vi "Acquire.vi"(5 "Weight Port":refnum<visa-resource-name>, 6 "error in":errorcluster, 7 "GlobalData":T1, 8 "Calibration":variant, 9 "Salinity":refnum<k21>, 10 "Temperature":refnum<k21>, 11 "Pressure":refnum<k21>) -> (0 "Weight Port":refnum<visa-resource-name>, 1 "Salinity":refnum<k21>, 2 "Temperature":refnum<k21>, 3 "Pressure":refnum<k21>, 4 "error out":errorcluster)   [LabVIEW 2024]
uses:
  <vilib>/DAQmx/read.llb/DAQmx Read (Analog DBL 1Chan 1Samp).vi
  controls/GlobalData.ctl
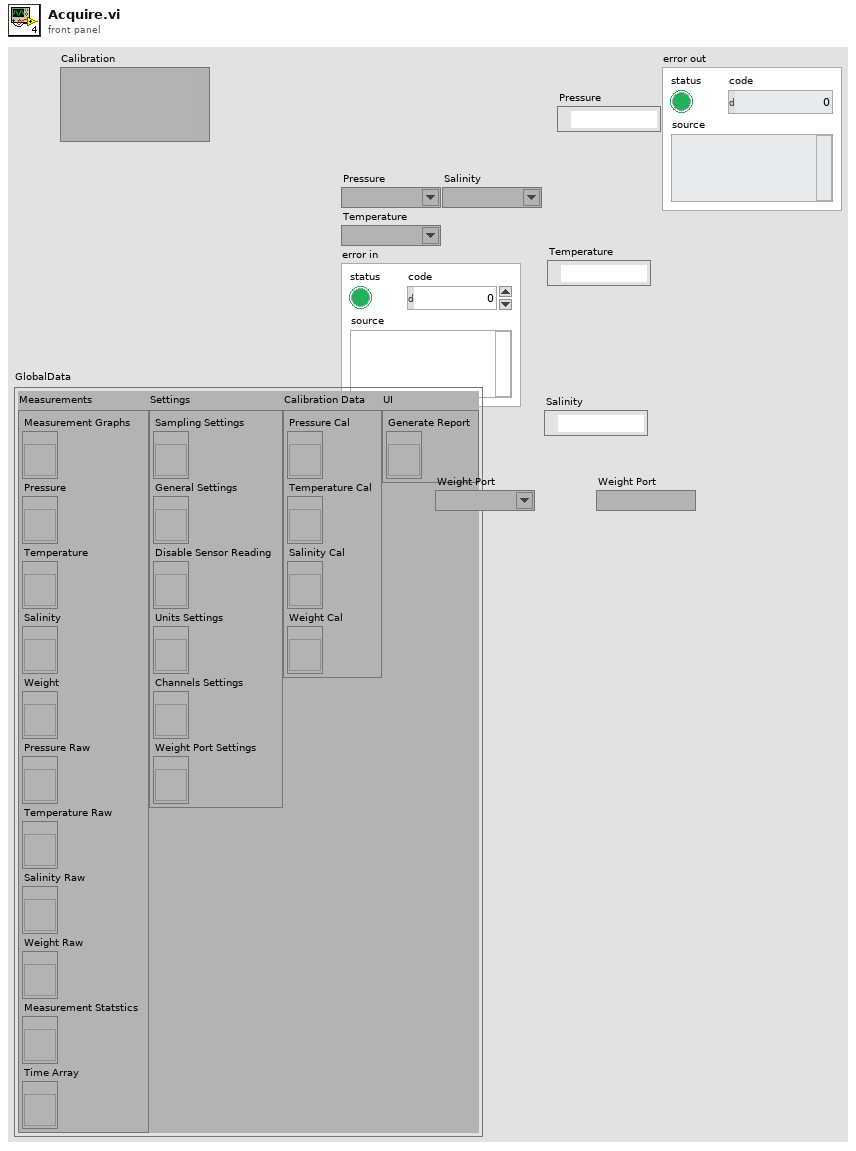
[diagram p1: front panel]
types:
  T1 = typedef "GlobalData.ctl" = cluster{"Measurements":cluster{"Measurement Graphs":refnum<vi>, "Pressure":refnum<vi>, "Temperature":refnum<vi>, "Salinity":refnum<vi>, "Weight":refnum<vi>, "Pressure Raw":refnum<vi>, "Temperature Raw":refnum<vi>, "Salinity Raw":refnum<vi>, "Weight Raw":refnum<vi>, "Measurement Statstics":refnum<vi>, "Time Array":refnum<vi>}, "Settings":cluster{"Sampling Settings":refnum<vi>, "General Settings":refnum<vi>, "Disable Sensor Reading":refnum<vi>, "Units Settings":refnum<vi>, "Channels Settings":refnum<vi>, "Weight Port Settings":refnum<vi>}, "Calibration Data":cluster{"Pressure Cal":refnum<vi>, "Temperature Cal":refnum<vi>, "Salinity Cal":refnum<vi>, "Weight Cal":refnum<vi>}, "UI":cluster{"Generate Report":refnum<vi>}}
  T2 = typedef "Units.ctl" = cluster{"Pressure":enum16{"PSI", "Bar", "atm", "Pa"}, "Temperature":enum16{"C", "K", "F"}, "Salinity":enum16{"ppm", "ppt", "PSU"}, "Weight":enum16{"Kg", "g", "oz", "ib"}}
  T3 = cluster{"C (Y-Intercept)":dbl, "M (Gradient)":dbl}
  T4 = cluster{"Pressure":dbl[], "Temperature":dbl[], "Salinity":dbl[], "Weight":dbl[]}
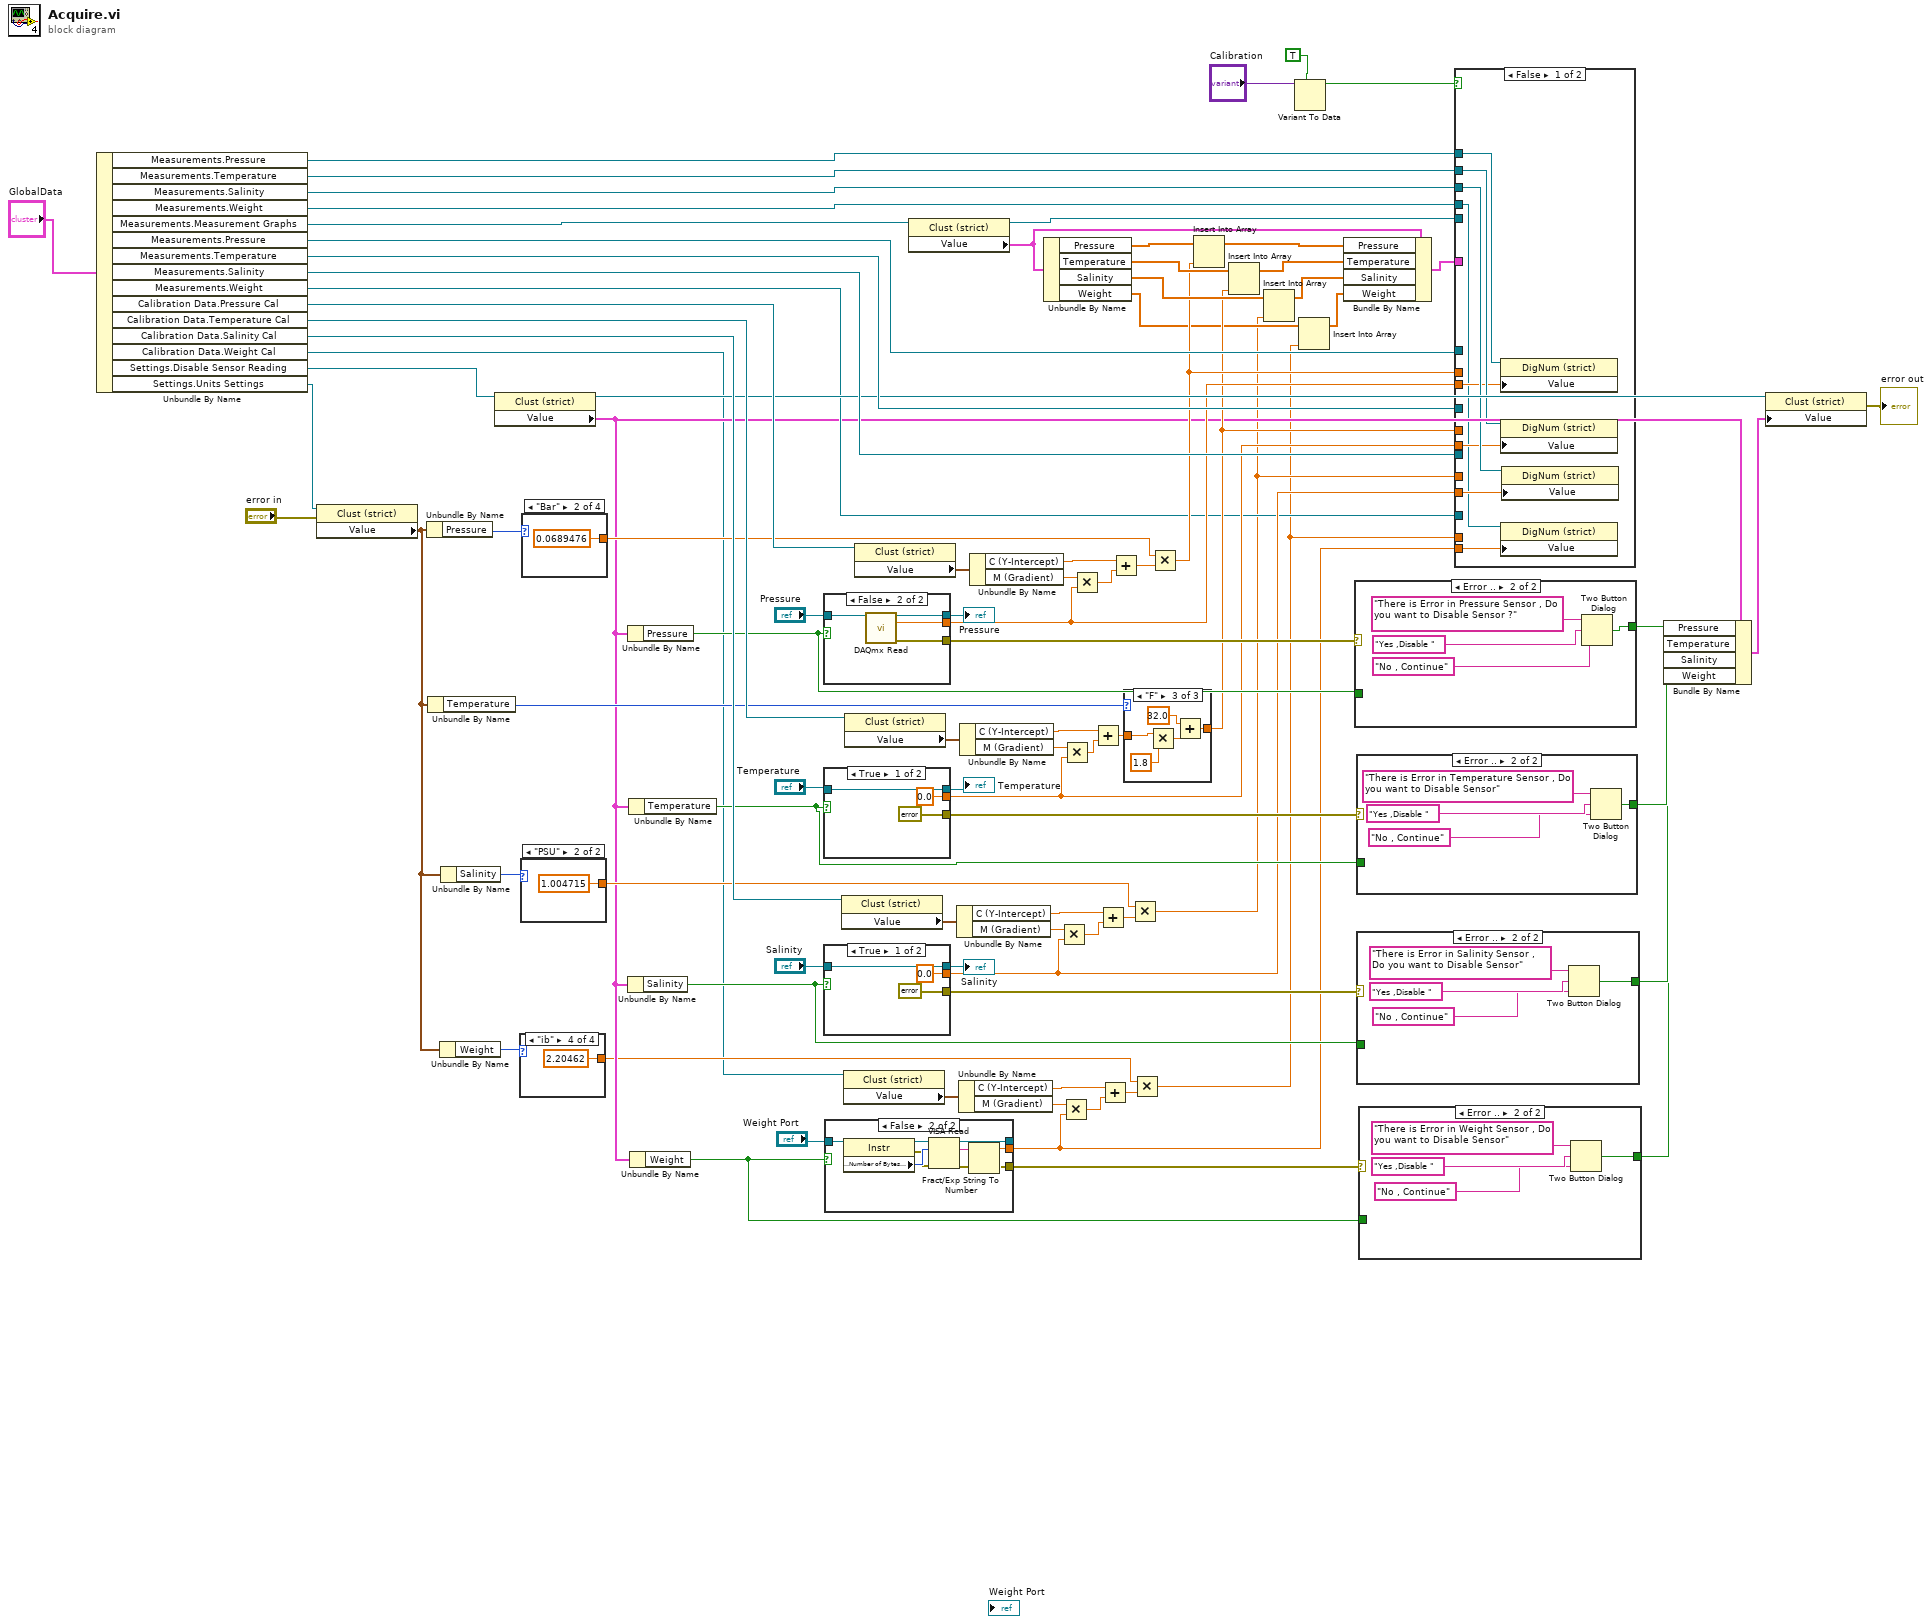
[diagram p0: block diagram]
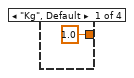
[diagram p2: hidden frame]
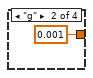
[diagram p3: hidden frame]
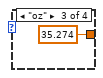
[diagram p4: hidden frame]
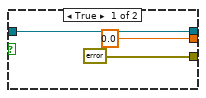
[diagram p6: hidden frame]
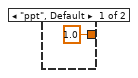
[diagram p7: hidden frame]
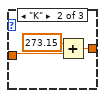
[diagram p9: hidden frame]
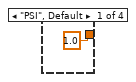
[diagram p10: hidden frame]
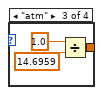
[diagram p11: hidden frame]
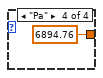
[diagram p12: hidden frame]
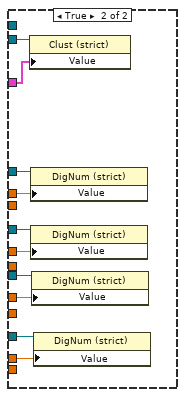
[diagram p13: hidden frame]
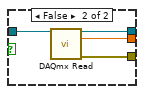
[diagram p16: hidden frame]
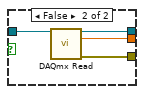
[diagram p17: hidden frame]
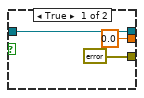
[diagram p18: hidden frame]
diagram:
  n1 = Unbundle By Name("GlobalData") -> ("Measurements.Pressure"=w45:refnum<vi>, "Measurements.Temperature"=w44:refnum<vi>, "Measurements.Salinity"=w43:refnum<vi>, "Measurements.Weight"=w1:refnum<vi>, "Measurements.Measurement Graphs"=w88:refnum<vi>, "Measurements.Pressure"=w79:refnum<vi>, "Measurements.Temperature"=w78:refnum<vi>, "Measurements.Salinity"=w77:refnum<vi>, "Measurements.Weight"=w18:refnum<vi>, "Calibration Data.Pressure Cal"=w72:refnum<vi>, "Calibration Data.Temperature Cal"=w63:refnum<vi>, "Calibration Data.Salinity Cal"=w62:refnum<vi>, "Calibration Data.Weight Cal"=w8:refnum<vi>, "Settings.Disable Sensor Reading"=w60:refnum<vi>, "Settings.Units Settings"=w38:refnum<vi>)
  n2 = property class="Clust (strict)"(reference=w38, error in="error in") -> ("Value"=w10:T2)  [unwired: 2 out]
  n3 = Unbundle By Name(w10) -> ("Pressure"=w34:enum16{"PSI", "Bar", "atm", "Pa"})
  n4 = Unbundle By Name(w10) -> ("Temperature"=w32:enum16{"C", "K", "F"})
  n5 = Unbundle By Name(w10) -> ("Weight"=w11:enum16{"Kg", "g", "oz", "ib"})
  n6 = Unbundle By Name(w10) -> ("Salinity"=w31:enum16{"ppm", "ppt", "PSU"})
  n7 = property class="Clust (strict)"(reference=w60) -> (reference out=w55:refnum<vi>, "Value"=w12:cluster{"Daq":bool, "RS232":bool})  [unwired: 1 in, 1 out]
  n8 = case shown="\"ib\"" w11 {
    tunnel: [1.0 ("C (Y-Intercept)") 0.001 ("C (Y-Intercept)") 35.274 ("C (Y-Intercept)") 2.20462 ("C (Y-Intercept)")] -> w9
    frame "Kg", Default {
    }
    frame "g" {
    }
    frame "oz" {
    }
    frame "ib" {
    }
  }
  n9 = case shown="\"PSU\"" w31 {
    tunnel: [1.0 ("C (Y-Intercept)") 1.004715 ("C (Y-Intercept)")] -> w30
    frame "ppt", Default {
    }
    frame "PSU" {
    }
  }
  n10 = case shown="\"Bar\"" w34 {
    tunnel: [1.0 ("C (Y-Intercept)") 0.0689476 ("C (Y-Intercept)") w101 6894.76 ("C (Y-Intercept)")] -> w33
    frame "PSI", Default {
    }
    frame "Bar" {
    }
    frame "atm" {
      n11 = Divide(x=1.0, y=14.6959) -> (x/y=w101:dbl)
    }
    frame "Pa" {
    }
  }
  n12 = Unbundle By Name(w12) -> ("Pressure"=w51:bool)
  n13 = Unbundle By Name(w12) -> ("Salinity"=w46:bool)
  n14 = Unbundle By Name(w12) -> ("Temperature"=w47:bool)
  n15 = Unbundle By Name(w12) -> ("Weight"=w5:bool)
  n16 = case shown="False" w51 {
    tunnel: [w105 w109] -> w90
    tunnel: "Pressure" -> [w105 w108]
    tunnel: [0.0 ("data") w107] -> w42
    tunnel: [errorcluster {"status"=FALSE, "code"=0, "source"=""} ("error out") w106] -> w61
    frame True {
    }
    frame False {
      n17 = call-poly <vilib>:"DAQmx Read.vi"("task/channels in"=w108) -> ("task out"=w109:refnum<k21>, "data"=w107:dbl, "error out"=w106:errorcluster)  [unwired: 12 in]
    }
  }
  "Pressure" <- w90
  n18 = case shown="True" w47 {
    tunnel: [w112 w116] -> w59
    tunnel: "Temperature" -> [w112 w115]
    tunnel: [0.0 ("data") w114] -> w41
    tunnel: [errorcluster {"status"=FALSE, "code"=0, "source"=""} ("error out") w113] -> w53
    frame True {
    }
    frame False {
      n19 = call-poly <vilib>:"DAQmx Read.vi"("task/channels in"=w115) -> ("task out"=w116:refnum<k21>, "data"=w114:dbl, "error out"=w113:errorcluster)  [unwired: 12 in]
    }
  }
  "Temperature" <- w59
  n20 = case shown="True" w46 {
    tunnel: [w119 w123] -> w58
    tunnel: "Salinity" -> [w119 w122]
    tunnel: [0.0 ("data") w121] -> w40
    tunnel: [errorcluster {"status"=FALSE, "code"=0, "source"=""} ("error out") w120] -> w52
    frame True {
    }
    frame False {
      n21 = call-poly <vilib>:"DAQmx Read.vi"("task/channels in"=w122) -> ("task out"=w123:refnum<k21>, "data"=w121:dbl, "error out"=w120:errorcluster)  [unwired: 12 in]
    }
  }
  "Salinity" <- w58
  n22 = case shown="False" w5 {
    tunnel: [w126 w130] -> _
    tunnel: "Weight Port" -> [w126 w132]
    tunnel: [0.0 ("data") w129] -> w2
    tunnel: [errorcluster {"status"=FALSE, "code"=0, "source"=""} ("error out") w128] -> w6
    frame True {
    }
    frame False {
      n23 = property class="Instr"(reference=w132) -> (reference out=w131:refnum<visa-resource-name>, error out=w127:errorcluster, "Serial Settings:Number of Bytes at Serial Port"=w133:u32)  [unwired: 1 in]
      n24 = VISA Read(VISA resource name=w131, byte count=w133, error in (no error)=w127) -> (VISA resource name out=w130:refnum<visa-resource-name>, read buffer=w134:string, error out=w128:errorcluster)  [unwired: 1 out]
      n25 = Fract/Exp String To Number(string=w134) -> (number=w129:dbl)  [unwired: 3 in, 1 out]
    }
  }
  n26 = property class="Clust (strict)"(reference=w62) -> ("Value"=w67:T3)  [unwired: 1 in, 2 out]
  n27 = property class="Clust (strict)"(reference=w8) -> ("Value"=w13:T3)  [unwired: 1 in, 2 out]
  n28 = property class="Clust (strict)"(reference=w63) -> ("Value"=w68:T3)  [unwired: 1 in, 2 out]
  n29 = property class="Clust (strict)"(reference=w72) -> ("Value"=w76:T3)  [unwired: 1 in, 2 out]
  n30 = property class="Clust (strict)"(reference=w88) -> (reference out=w80:refnum<vi>, "Value"=w85:T4)  [unwired: 1 in, 1 out]
  n31 = Unbundle By Name(w67) -> ("C (Y-Intercept)"=w64:dbl, "M (Gradient)"=w66:dbl)
  n32 = Unbundle By Name(w13) -> ("C (Y-Intercept)"=w16:dbl, "M (Gradient)"=w14:dbl)
  n33 = Unbundle By Name(w68) -> ("C (Y-Intercept)"=w71:dbl, "M (Gradient)"=w69:dbl)
  n34 = Unbundle By Name(w76) -> ("C (Y-Intercept)"=w73:dbl, "M (Gradient)"=w75:dbl)
  n35 = Unbundle By Name(w85) -> ("Pressure"=w87:dbl[], "Temperature"=w83:dbl[], "Salinity"=w82:dbl[], "Weight"=w20:dbl[])
  n36 = Multiply(x=w66, y=w40) -> (x*y=w65:dbl)
  n37 = Multiply(x=w14, y=w2) -> (x*y=w15:dbl)
  n38 = Multiply(x=w69, y=w41) -> (x*y=w70:dbl)
  n39 = Multiply(x=w75, y=w42) -> (x*y=w74:dbl)
  n40 = Add(x=w71, y=w70) -> (x+y=w28:dbl)
  n41 = Add(x=w64, y=w65) -> (x+y=w35:dbl)
  n42 = Add(x=w16, y=w15) -> (x+y=w17:dbl)
  n43 = Add(x=w73, y=w74) -> (x+y=w37:dbl)
  n44 = case shown="\"F\"" w32 {
    tunnel: [w135 w138 w143] -> w29
    tunnel: w28 -> [w135 w137 w140]
    frame "C", Default {
    }
    frame "K" {
      n45 = Add(x=273.15, y=w137) -> (x+y=w138:dbl)
    }
    frame "F" {
      n46 = Multiply(x=w140, y=1.8 ("x")) -> (x*y=w141:dbl)
      n47 = Add(x=32.0, y=w141) -> (x+y=w143:dbl)
    }
  }
  n48 = Multiply(x=w30, y=w35) -> (x*y=w7:dbl)
  n49 = Multiply(x=w9, y=w17) -> (x*y=w3:dbl)
  n50 = Multiply(x=w33, y=w37) -> (x*y=w36:dbl)
  n51 = Insert Into Array(array=w87, new element=w36) -> (w86:dbl[])  [unwired: 1 in]
  n52 = Insert Into Array(array=w83, new element=w29) -> (w84:dbl[])  [unwired: 1 in]
  n53 = Insert Into Array(array=w82, new element=w7) -> (w22:dbl[])  [unwired: 1 in]
  n54 = Variant To Data(type=TRUE ("Calibration"), Variant="Calibration") -> (data=w24:bool)  [unwired: 1 in, 1 out]
  n55 = Insert Into Array(array=w20, new element=w3) -> (w21:dbl[])  [unwired: 1 in]
  n56 = Bundle By Name(cluster=w85, "Pressure"=w86, "Temperature"=w84, "Salinity"=w22, "Weight"=w21) -> (w81:T4)
  n57 = case shown="Error .." w61 {
    tunnel: w51 -> [w144 _]
    tunnel: [w144 w145] -> w50
    frame No Error {
    }
    frame Error {
      n58 = Two Button Dialog(message="There is Error in Pressure Sensor , Do you want to Disable Sensor ?", 1:"No , Continue" ("F button name (\"Cancel\")"), 2:"Yes ,Disable " ("T button name (\"OK\")")) -> (T button?=w145:bool)
    }
  }
  n59 = case shown="Error .." w53 {
    tunnel: [w149 w150] -> w49
    tunnel: w47 -> [w149 _]
    frame No Error {
    }
    frame Error {
      n60 = Two Button Dialog(message="There is Error in Temperature Sensor , Do you want to Disable Sensor", 1:"No , Continue" ("F button name (\"Cancel\")"), 2:"Yes ,Disable " ("T button name (\"OK\")")) -> (T button?=w150:bool)
    }
  }
  n61 = case shown="Error .." w52 {
    tunnel: [w154 w155] -> w48
    tunnel: w46 -> [w154 _]
    frame No Error {
    }
    frame Error {
      n62 = Two Button Dialog(message="There is Error in Salinity Sensor , Do you want to Disable Sensor", 1:"No , Continue" ("F button name (\"Cancel\")"), 2:"Yes ,Disable " ("T button name (\"OK\")")) -> (T button?=w155:bool)
    }
  }
  n63 = case shown="Error .." w6 {
    tunnel: [w159 w160] -> w4
    tunnel: w5 -> [w159 _]
    frame No Error {
    }
    frame Error {
      n64 = Two Button Dialog(message="There is Error in Weight Sensor , Do you want to Disable Sensor", 1:"No , Continue" ("F button name (\"Cancel\")"), 2:"Yes ,Disable " ("T button name (\"OK\")")) -> (T button?=w160:bool)
    }
  }
  n65 = case shown="False" w24 {
    tunnel: w81 -> [_ w181]
    tunnel: w80 -> [_ w180]
    tunnel: w79 -> [_ w179]
    tunnel: w78 -> [_ w178]
    tunnel: w77 -> [_ w177]
    tunnel: w36 -> [_ w176]
    tunnel: w29 -> [_ w175]
    tunnel: w7 -> [_ w174]
    tunnel: w45 -> [w171 _]
    tunnel: w44 -> [w170 _]
    tunnel: w43 -> [w169 _]
    tunnel: w42 -> [w168 _]
    tunnel: w41 -> [w167 _]
    tunnel: w40 -> [w166 _]
    tunnel: w18 -> [_ w173]
    tunnel: w3 -> [_ w172]
    tunnel: w2 -> [w165 _]
    tunnel: w1 -> [w164 _]
    frame False {
      n66 = property class="DigNum (strict)"(reference=w171, "Value"=w168) -> ()  [unwired: 1 in, 2 out]
      n67 = property class="DigNum (strict)"(reference=w170, "Value"=w167) -> ()  [unwired: 1 in, 2 out]
      n68 = property class="DigNum (strict)"(reference=w164, "Value"=w165) -> ()  [unwired: 1 in, 2 out]
      n69 = property class="DigNum (strict)"(reference=w169, "Value"=w166) -> ()  [unwired: 1 in, 2 out]
    }
    frame True {
      n70 = property class="Clust (strict)"(reference=w180, "Value"=w181) -> ()  [unwired: 1 in, 2 out]
      n71 = property class="DigNum (strict)"(reference=w179, "Value"=w176) -> ()  [unwired: 1 in, 2 out]
      n72 = property class="DigNum (strict)"(reference=w178, "Value"=w175) -> ()  [unwired: 1 in, 2 out]
      n73 = property class="DigNum (strict)"(reference=w177, "Value"=w174) -> ()  [unwired: 1 in, 2 out]
      n74 = property class="DigNum (strict)"(reference=w173, "Value"=w172) -> ()  [unwired: 1 in, 2 out]
    }
  }
  n75 = Bundle By Name(cluster=w12, "Pressure"=w50, "Temperature"=w49, "Salinity"=w48, "Weight"=w4) -> (w54:cluster{"Daq":bool, "RS232":bool})
  n76 = property class="Clust (strict)"(reference=w55, "Value"=w54) -> (error out=→"error out":errorcluster)  [unwired: 1 in, 1 out]
